vi "Degrees To Ticks.vi"(11 "degrees":dbl) -> (3 "ticks":dbl)   [LabVIEW 2020]
doc: "unit conversion: degrees --> ticks (multiplying)"
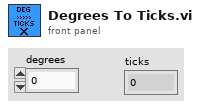
[diagram p1: front panel]
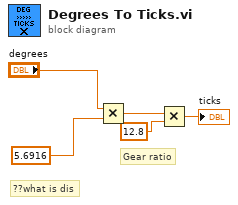
[diagram p0: block diagram]
diagram:
  # "??what is dis"
  # "Gear ratio"
  n1 = Multiply(x="degrees", y=5.6916 ("scale factor")) -> (x*y=w5:dbl)
  n2 = Multiply(x=w5, y=12.8) -> (x*y=→"ticks":dbl)
